vi "Coords to chart(new).vi"(1 "DataLine":string[](array[string]), 2 "options":i16(ring) items=["tel coords", "guidage", "notes"], 3 "Tableau entrant":string[][](table)) -> (0 "historique":string[][](table))   [LabVIEW 2019]
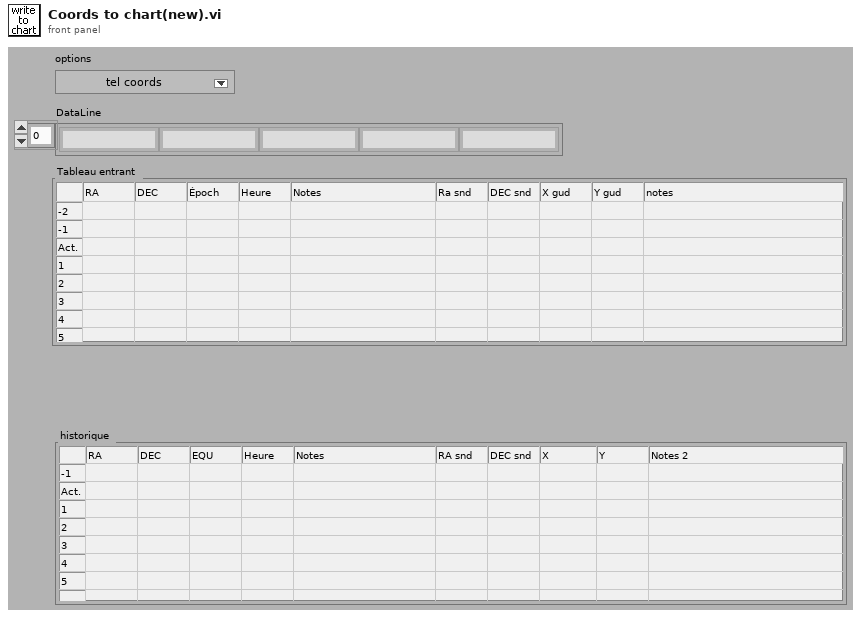
[diagram p1: front panel]
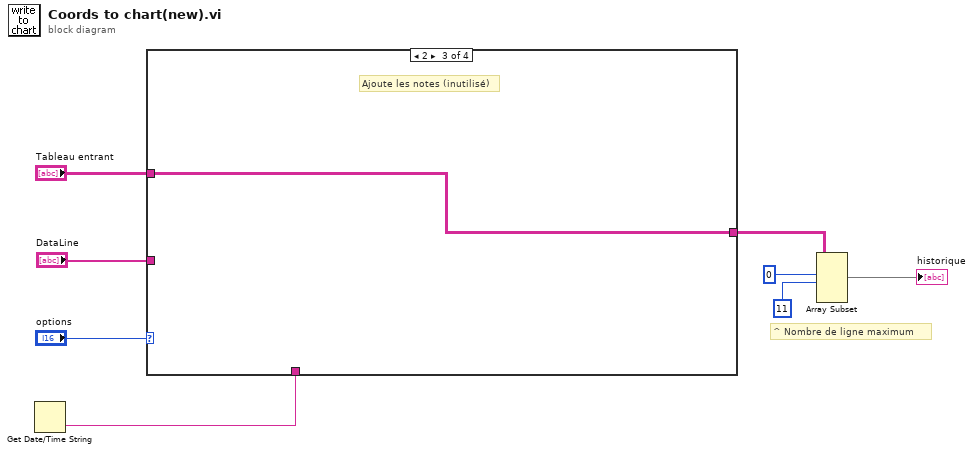
[diagram p0: block diagram]
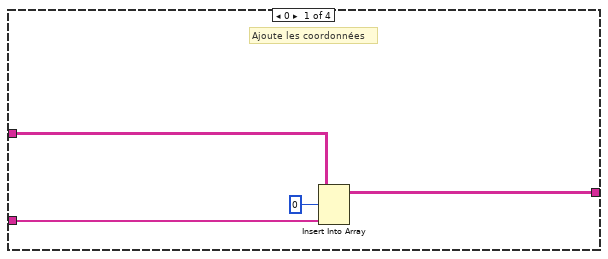
[diagram p2: hidden frame]
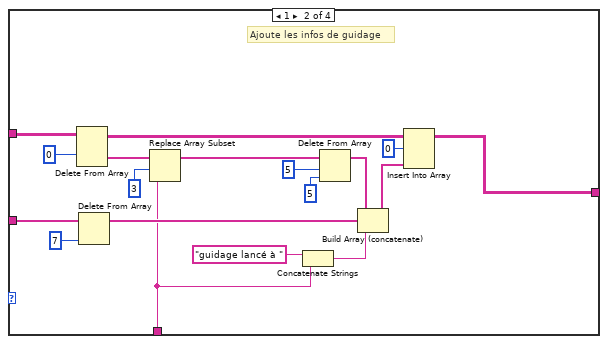
[diagram p3: hidden frame]
diagram:
  # "^ Nombre de ligne maximum"
  n1 = Get Date/Time String() -> (time string=w1:string)  [unwired: 3 in, 1 out]
  n2 = case shown="2" "options" {
    tunnel: "Tableau entrant" -> [w11 w29 w31 w32]
    tunnel: [w10 w30 w31 w32] -> w3
    tunnel: "DataLine" -> [w9 w27 _ _]
    tunnel: w1 -> [_ w14 _ _]
    frame 0 {
      # "Ajoute les coordonnées"
      n3 = Insert Into Array(array=w11, index (row)=0 ("indice (ligne)"), new element=w9) -> (w10:string[][])  [unwired: 1 in]
    }
    frame 1 {
      # "Ajoute les infos de guidage"
      n4 = Delete From Array(array=w29, index (row)=0) -> (deleted portion=w18:string[], array with subset deleted=w19:string[][])  [unwired: 2 in]
      n5 = Delete From Array(array=w27, index=7) -> (array with subset deleted=w25:string[])  [unwired: 1 in, 1 out]
      n6 = Replace Array Subset(array=w18, new element=w14, index=3 ("disabled index (col)")) -> (w17:string[])
      n7 = Concatenate Strings("guidage lancé à ", w14) -> (w13:string)
      n8 = Delete From Array(array=w17, length=5, index=5) -> (array with subset deleted=w23:string[])  [unwired: 1 out]
      n9 = Build Array (concatenate)(w23, w25, w13) -> (w24:string[])
      n10 = Insert Into Array(array=w19, index (row)=0, new element=w24) -> (w30:string[][])  [unwired: 1 in]
    }
    frame 2 {
      # "Ajoute les notes (inutilisé)"
    }
    frame -1, Default {
    }
  }
  n11 = Array Subset(array=w3, index (row)=0 ("index"), length (row)=11 ("length")) -> (→"historique":string[][])  [unwired: 2 in]
